vi "GA_Find_NumberofScheduled_Jobs_On_Particular_Machine.vi"(10 "Machine No":i32, 11 "Job Schedule on Machines":i32[][](array[numeric])) -> (3 "Number of Scheduled Jobs On Current Machine":i32)   [LabVIEW 2013, in "GA.lvclass"]
uses:
  GA.lvclass
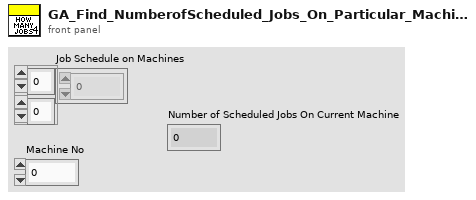
[diagram p1: front panel]
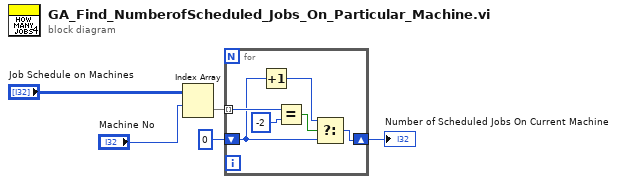
[diagram p0: block diagram]
diagram:
  n1 = Index Array(array="Job Schedule on Machines", index (row)="Machine No") -> (element=w3:i32[])  [unwired: 1 in]
  n2 = for {
    tunnel: w3 -> [w11] mode=indexing
    shift-right: [w7] -> w1
    shift-left: 0 -> [w6]
    n3 = Increment(x=w6) -> (x+1=w8:i32)
    n4 = Equal?(x=w11, y=-2) -> (x = y?=w9:bool)
    n5 = Select(t=w8, s=w9, f=w6) -> (s? t:f=w7:i32)
  }
  "Number of Scheduled Jobs On Current Machine" <- w1
